vi "6_Signals_stimulus_clean.vi"() -> ()   [LabVIEW 2017]
panel:
  out "Array":i16[][](array[numeric])
  in  "Delayed 3.75 ns":bool
  in  "Delayed 2.5 ns":bool
  out "Read A Ready":i16[](graph)
  out "Read B Ready":i16[](graph)
  out "sample":i32[](graph)
  out "pixel value 2":i32[](graph)
  in  "zero signal":bool
  in  "scale":dbl
  in  "Delayed 1.25ns":bool
  in  "cycles":i32
  in  "Offset":dbl
  in  "expdiv":sgl
  in  "ArraySize":i32=100
  out "Signal Generated":dbl[](graph)
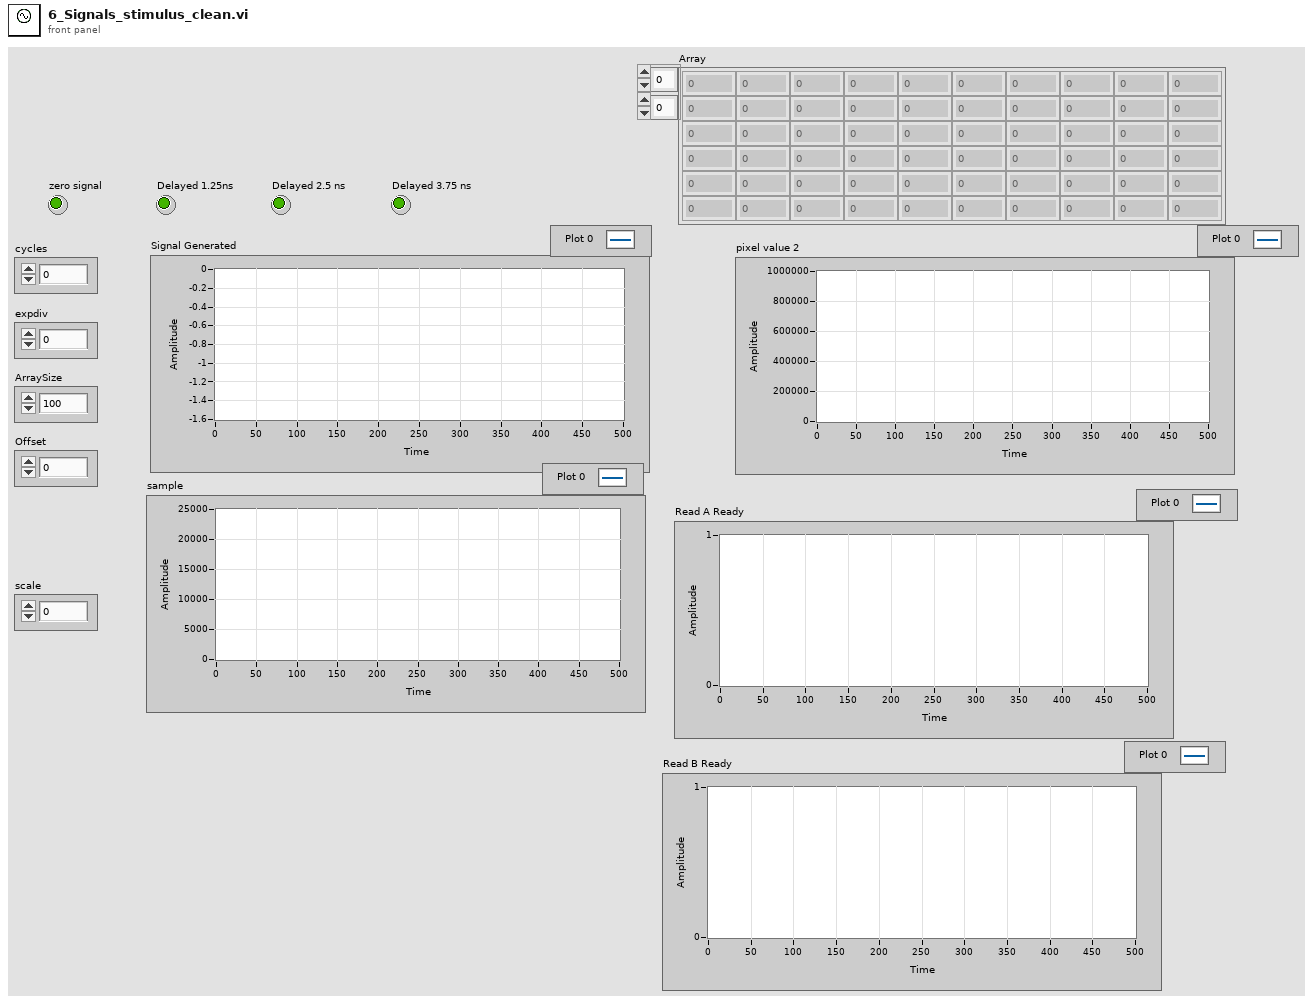
[diagram p1: front panel]
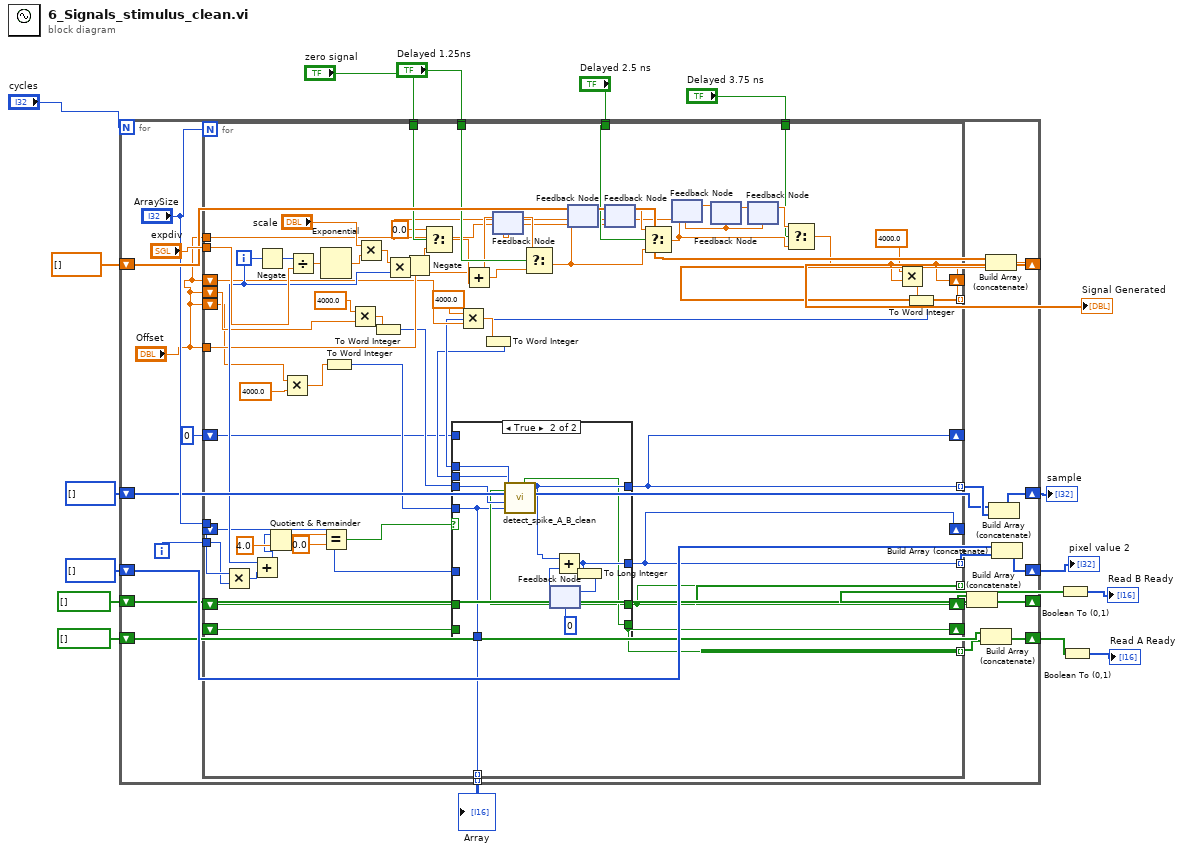
[diagram p0: block diagram]
diagram:
  n1 = for {
    N: "cycles" -> [_]
    shift-right: [w41] -> w17
    shift-left: dbl[] [] -> [w40]
    tunnel: "Delayed 1.25ns" -> [w38]
    tunnel: "zero signal" -> [w37]
    shift-right: [w34] -> w12
    shift-left: i32[] [] -> [w33]
    shift-right: [w31] -> w10
    shift-left: i32[] [] -> [w30]
    shift-right: [w29] -> w5
    shift-left: bool[] [] -> [w28]
    shift-right: [w27] -> w7
    shift-left: bool[] [] -> [w25]
    tunnel: "Delayed 2.5 ns" -> [w22]
    tunnel: "Delayed 3.75 ns" -> [w21]
    tunnel: [w19] -> w1 mode=indexing
    i -> [w39]
    n2 = for {
      N: "ArraySize" -> [_]
      tunnel: "expdiv" -> [w100]
      tunnel: [w45] -> w42 mode=indexing
      shift-right: [w45] -> _
      shift-left: "Offset" -> [w77]
      shift-left: "Offset" -> [w74]
      tunnel: w39 -> [w92]
      tunnel: "ArraySize" -> [w96]
      tunnel: w38 -> [w91]
      tunnel: w37 -> [w86]
      tunnel: "Offset" -> [w82]
      shift-left: "Offset" -> [w71]
      shift-right: [w65] -> _
      shift-left: 0 ("Numeric") -> [w64]
      tunnel: [w65] -> w32 mode=indexing
      tunnel: [w63] -> w35 mode=indexing
      shift-right: [w63] -> _
      shift-left: _ -> [w62]
      shift-right: [w60] -> _
      shift-left: _ -> [w61]
      tunnel: [w60] -> w26 mode=indexing
      shift-right: [w58] -> _
      shift-left: _ -> [w59]
      tunnel: [w58] -> w24 mode=indexing
      tunnel: w22 -> [w51]
      tunnel: w21 -> [w48]
      tunnel: "Offset" -> [w47]
      tunnel: [w46] -> w19 mode=indexing
      i -> [w94]
      n3 = Multiply(x=w96, y=w92) -> (x*y=w95:i32)
      n4 = Add(x=w94, y=w95) -> (x+y=w93:i32)
      n5 = Negate(x=w94) -> (-x=w101:i32)
      n6 = Quotient & Remainder(x=w93, y=4.0) -> (x-y*floor(x/y)=w99:dbl)  [unwired: 1 out]
      n7 = Multiply(x=w71, y=4000.0 ("x")) -> (x*y=w70:dbl)
      n8 = Divide(x=w101, y=w100) -> (x/y=w102:sgl)
      n9 = Exponential(1:w102) -> (0:w87:sgl)
      n10 = Equal?(x=w99, y=0.0) -> (x = y?=w57:bool)
      n11 = To Word Integer(number=w70) -> (16bit integer=w66:i16)
      n12 = Multiply(x=4000.0, y=w74) -> (x*y=w73:dbl)
      n13 = Multiply(x="scale", y=w87) -> (x*y=w88:dbl)
      n14 = To Word Integer(number=w73) -> (16bit integer=w67:i16)
      n15 = Multiply(x=w88, y=w94) -> (x*y=w85:dbl)
      n16 = Negate(x=w85) -> (-x=w44:dbl)
      n17 = Select(t=0.0, s=w86, f=w44) -> (s? t:f=w84:dbl)
      n18 = Multiply(x=4000.0, y=w77) -> (x*y=w76:dbl)
      n19 = Add(x=w82, y=w84) -> (x+y=w81:dbl)
      n20 = To Word Integer(number=w76) -> (16bit integer=w68:i16)
      n21 = feedback-in #1(w81) -> ()
      n22 = feedback #1(w47) -> (w90:dbl)
      n23 = Select(t=w90, s=w91, f=w81) -> (s? t:f=w49:dbl)
      n24 = feedback #2(w47) -> (w50:dbl)
      n25 = feedback-in #2(w49) -> ()
      n26 = feedback #3(w47) -> (w56:dbl)
      n27 = feedback-in #3(w50) -> ()
      n28 = Select(t=w56, s=w51, f=w49) -> (s? t:f=w52:dbl)
      n29 = feedback #4(w47) -> (w53:dbl)
      n30 = feedback-in #4(w52) -> ()
      n31 = feedback #5(w47) -> (w54:dbl)
      n32 = feedback-in #5(w53) -> ()
      n33 = feedback #6(w47) -> (w55:dbl)
      n34 = feedback-in #6(w54) -> ()
      n35 = Select(t=w55, s=w48, f=w52) -> (s? t:f=w45:dbl)
      n36 = Multiply(x=4000.0, y=w45) -> (x*y=w79:dbl)
      n37 = To Word Integer(number=w79) -> (16bit integer=w69:i16)
      n38 = case shown="True" w57 {
        tunnel: w69 -> [_ w118]
        tunnel: w68 -> [_ w117]
        tunnel: w67 -> [_ w116]
        tunnel: [w106 w112] -> w63
        tunnel: [w107 w111] -> w65
        tunnel: w66 -> [w103 w108]
        tunnel: w64 -> [w107 _]
        tunnel: w62 -> [w106 _]
        tunnel: w61 -> [w105 _]
        tunnel: [w105 w110] -> w60
        tunnel: [w104 w109] -> w58
        tunnel: w59 -> [w104 _]
        tunnel: [w103 w108] -> w46
        frame False {
        }
        frame True {
          n39 = call "detect_spike_A_B_clean.vi"("IO Module\\AI 1 Data N-3"=w108, "IO Module\\AI 1 Data N-2"=w116, "IO Module\\AI 1 Data N-1"=w117, "IO Module\\AI 1 Data N"=w118) -> ("Numeric"=w111:i32, "Read Ready A"=w110:bool, "Read Ready B"=w109:bool)  [unwired: 5 in]
          n40 = feedback #7(0) -> (w114:i32)
          n41 = Add(x=w111, y=w114) -> (x+y=w112:i32)
          n42 = To Long Integer(number=w112) -> (32bit integer=w113:i32)
          n43 = feedback-in #7(w113) -> ()
        }
      }
    }
    n44 = Build Array (concatenate)(w25, w24) -> (w27:bool[])
    n45 = Build Array (concatenate)(w28, w26) -> (w29:bool[])
    n46 = Build Array (concatenate)(w40, w42) -> (w41:dbl[])
    n47 = Build Array (concatenate)(w30, w32) -> (w31:i32[])
    n48 = Build Array (concatenate)(w33, w35) -> (w34:i32[])
  }
  "Signal Generated" <- w17
  "pixel value 2" <- w12
  "sample" <- w10
  "Array" <- w1
  n49 = Boolean To (0,1)(Boolean=w7) -> (0, 1=→"Read B Ready":i16[])
  n50 = Boolean To (0,1)(Boolean=w5) -> (0, 1=→"Read A Ready":i16[])
